vi "Robot Global Data.vi"() -> ()   [LabVIEW 2020]
doc: "This global VI can contain as many global variables as you need. Place a control on the panel, give it a good name. To read or write to it from a VI, drag the icon to the diagram of that VI. You can also drag from the project. Click on the node to change which global you access. You shouldn't have multiple locations writing to a global or it will cause a race-condition."
uses:
  <vilib>/Rock Robotics/WPI/Camera/WPI_CameraImageSize.ctl
  <vilib>/Rock Robotics/WPI/DriverStation/WPI_DriverStationRobotMode2.ctl
panel:
  out "Grabber Motor Outtake 2":bool
  out "Grabber Motor Intake 2":bool
  out "AutoTDown":bool
  out "AutoTUp":bool
  out "Grabber Motor Outtake":bool
  out "Grabber Motor Intake":bool
  out "AEncoderTiltReset":bool
  out "EncoderTL":dbl
  out "EncoderTR":dbl
  out "HE Low On/Off":bool
  out "HE Hi On/Off":bool
  out "AEDownStop":bool
  out "AEUpStop":bool
  out "AutoOuttake":bool
  out "AutoIntake":bool
  out "AutoEDown":bool
  out "AutoEUp":bool
  out "EncoderER":dbl
  out "EncoderEL":dbl
  out "AEncoderElevatorReset":bool
  out "ADriveRotate":dbl
  out "ADriveStrafe":dbl
  out "ADriveFR":dbl
  out "J1 Button 03":bool
  out "J1 Button 12":bool
  out "J1 Button 11":bool
  out "J1 Button 10":bool
  out "J1 Button 09":bool
  out "J1 Button 08":bool
  out "J1 Button 07":bool
  out "J1 Button 06":bool
  out "J1 Button 05":bool
  out "J1 Button 04":bool
  out "J1 Button 02":bool
  out "J1 Trigger":bool
  out "J1 Throttle":dbl
  out "J1 Z-Axis":dbl
  out "J1 Y-Axis":dbl
  out "J1 X-Axis":dbl
  out "J0 Button 12":bool
  out "J0 Button 11":bool
  out "J0 Button 10":bool
  out "J0 Button 09":bool
  out "J0 Button 08":bool
  out "J0 Button 07":bool
  out "J0 Button 06":bool
  out "J0 Button 05":bool
  out "J0 Button 04":bool
  out "J0 Button 03":bool
  out "J0 Button 02":bool
  out "J0 Trigger":bool
  out "J0 Throttle":dbl
  out "J0 Z-Axis":dbl
  out "J0 Y-Axis":dbl
  out "J0 X-Axis":dbl
  in  "Robot Mode":T1
  in  "image size":T2=enum."320x240"
  in  "Enable Vision":bool
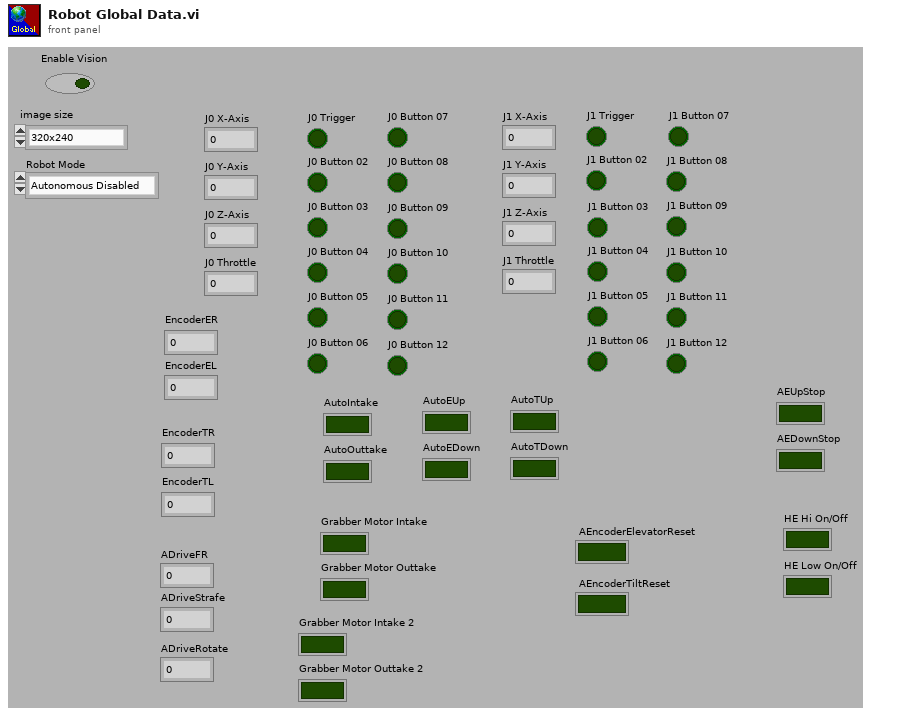
[diagram p1: front panel]
types:
  T1 = typedef "WPI_DriverStationRobotMode2.ctl" = enum16{"Autonomous Disabled", "Autonomous Enabled", "Teleop Disabled", "Teleop Enabled", "Disconnected", "Finish", "Test Disabled", "Test Enabled", "Emergency Stopped"}
  T2 = typedef "WPI_CameraImageSize.ctl" = enum16{"640x480", "320x240", "160x120", "Custom"}
diagram:
